vi "Destroy Bus Load Calculator.vi"(8 "error in (no error)":errorcluster, 11 "Load Calculator":refnum<class "CANBus_Load_Calculator.lvclass">) -> (0 "error out":errorcluster)   [LabVIEW 2018, in "NI-XNET Monitor Engine.lvlib" / "XNET-Bus-Load-Calculator.lvlib"]
uses:
  XNET-Bus-Load-Calculator.lvlib
  CANBus/CANBus_Load_Calculator.lvclass
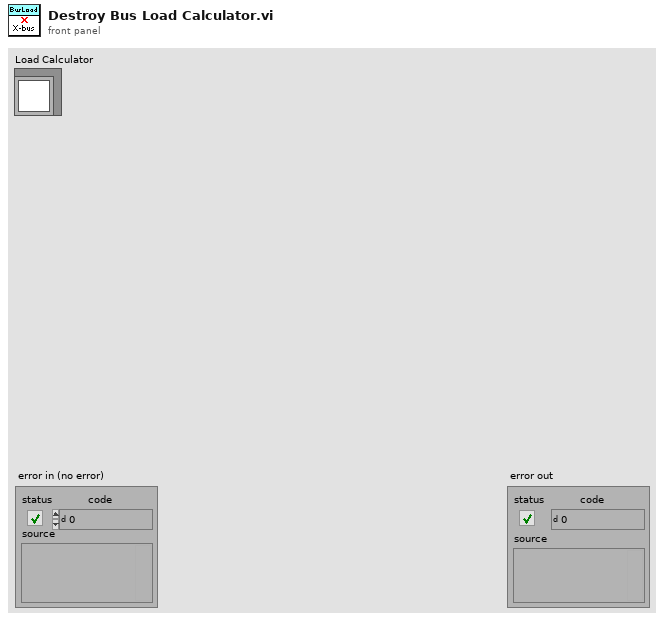
[diagram p1: front panel]
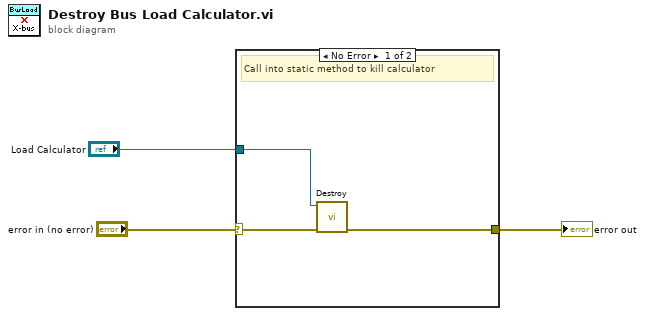
[diagram p0: block diagram]
diagram:
  n1 = case shown="No Error" "error in (no error)" {
    selector: "error in (no error)" -> [w6 w7]
    tunnel: [w4 w7] -> w2
    tunnel: "Load Calculator" -> [w5 _]
    frame No Error {
      # "Call into static method to kill calculator"
      n2 = call "Destroy.vi"("error in (no error)"=w6, "GenBus_Load_Calculator in"=w5) -> ("error out"=w4:errorcluster)  [unwired: 9 in]
    }
    frame Error {
    }
  }
  "error out" <- w2
